vi "Tenney_Main_Temperature_Changer.vi"(0 "Message Queues out":T2, 1 "Elapsed Time (min) Ref":refnum<vi>, 3 "Loop Count Ref":refnum<vi>, 5 "Debug":bool, 7 "Enable Arrays":bool=TRUE, 9 "Tenney Array":refnum<vi>, 11 "error in":errorcluster, 12 "Tenney IP Address":string="10.2.0.248", 13 "Connect Tenney Ref":refnum<vi>, 14 "Data Array":refnum<vi>) -> (15 "error out":errorcluster)   [LabVIEW 2023]
uses:
  Message Queue/All Message Queues.ctl
  Message Queue/Message Cluster.ctl
  Drivers/Tidal Engineering/Type Definitions/Tenney Environmental Chamber Data.ctl
  <vilib>/NI/Modbus Library/API/Master/Modbus Master.lvclass
  Drivers/Tidal Engineering/Type Definitions/Tenney Modbus Registers.ctl
  Drivers/Tidal Engineering/Type Definitions/Tenney Chamber Status.ctl
  controls/Tenney Temperature Limits.ctl
  Drivers/Viasala Indigo 520/Type Definitions/Viasala Indigo 520 Data.ctl
  Message Queue/Enqueue Message (Single).vi
  Message Queue/Tenney Message Queue.lvlib
panel:
  out "Connect Tenney Counter":dbl
  out "10 Minute Data Array Output":dbl[][](array[numeric])
  out "Elapsed Time (min)":dbl caption="Elapsed Time (s)"
  out "Set Chamber Status":dbl
  out "appended array":string[](array[string])
  out "Tenney Environmental Chamber Data Output":T1
  out "Humidity Counter":dbl
  out "Frequency Counter":dbl
  out "Temp Counter":dbl
  out "Loop Count":i32
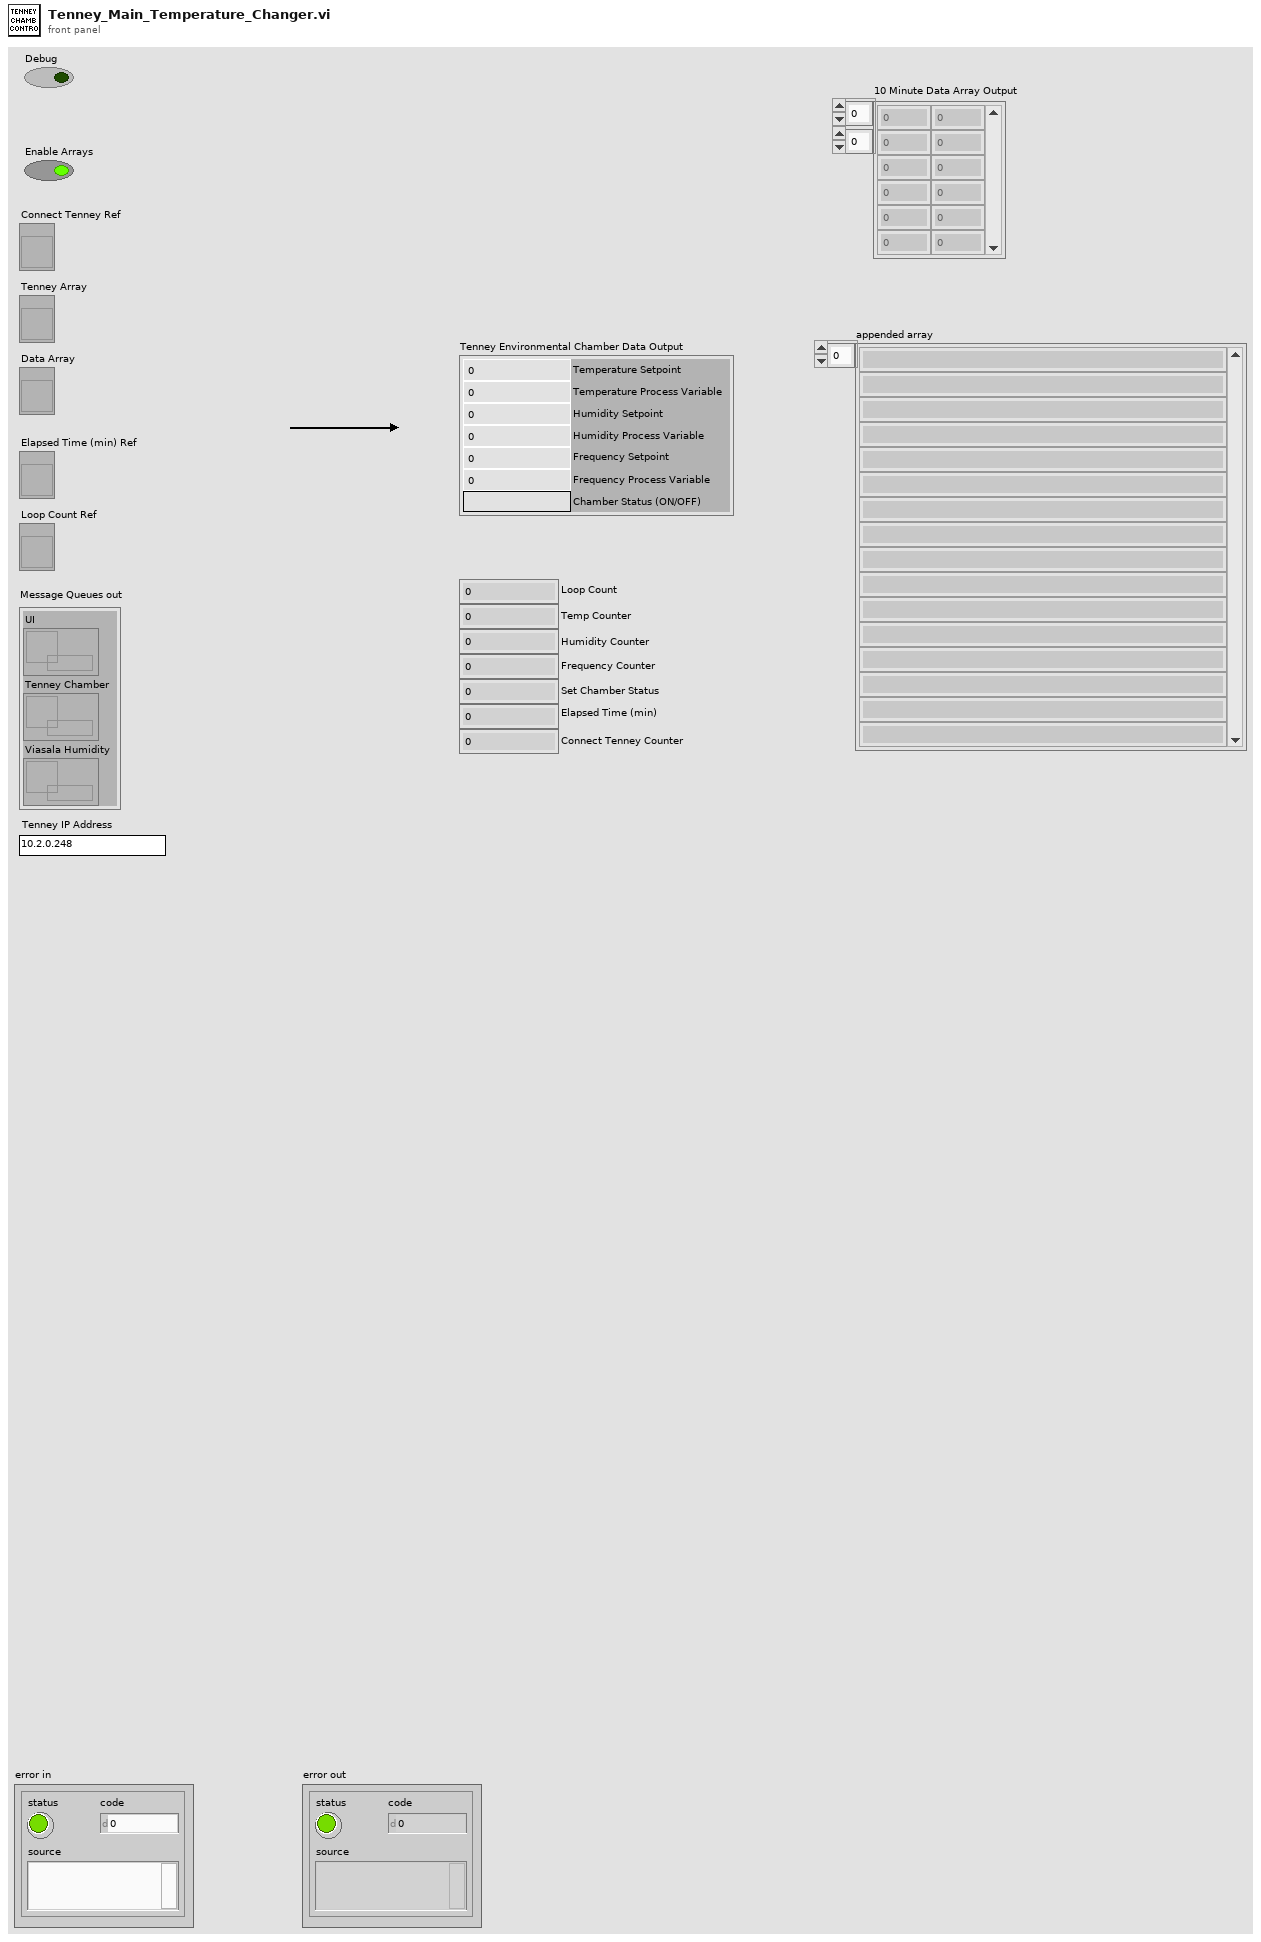
[diagram p1: front panel]
types:
  T1 = typedef "Tenney Environmental Chamber Data.ctl" = cluster{"Temperature Setpoint":dbl, "Temperature Process Variable":dbl, "Humidity Setpoint":dbl, "Humidity Process Variable":dbl, "Frequency Setpoint":dbl, "Frequency Process Variable":dbl, "Chamber Status (ON/OFF)":string}
  T2 = typedef "Tenney Message Queue.lvlib/All Message Queues.ctl" = cluster{"UI":refnum<queue>, "Tenney Chamber":refnum<queue>, "Viasala Humidity":refnum<queue>}
  T3 = typedef "Tenney Chamber Status.ctl" = enum16{"OFF", "ON"}
  T4 = typedef "Tenney Temperature Limits.ctl" = cluster{"Target Temperature Upper limit":dbl, "Target Temperature Lower limit":dbl, "Target Humidity Lower limit":dbl, "Target Humidity Upper limit":dbl, "Chamber Temperature Upper limit":dbl, "Chamber Temperature Lower limit":dbl, "Chamber Humidity Lower limit":dbl, "Chamber Humidity Upper limit":dbl, "Chamber Adjustment Increment (F)":dbl, "Chamber Adjustment Interval (Minutes)":dbl, "Chamber Adjustment Increment (%)":dbl, "Chamber Adjustment Interval Fast (Minutes)":dbl}
  T5 = typedef "Viasala Indigo 520 Data.ctl" = cluster{"Temperature Probe 1":dbl, "Humidity Probe 1":dbl, "Temperature Probe 2":dbl, "Humidity Probe 2":dbl}
  T6 = typedef "Tenney Modbus Registers.ctl" = u16
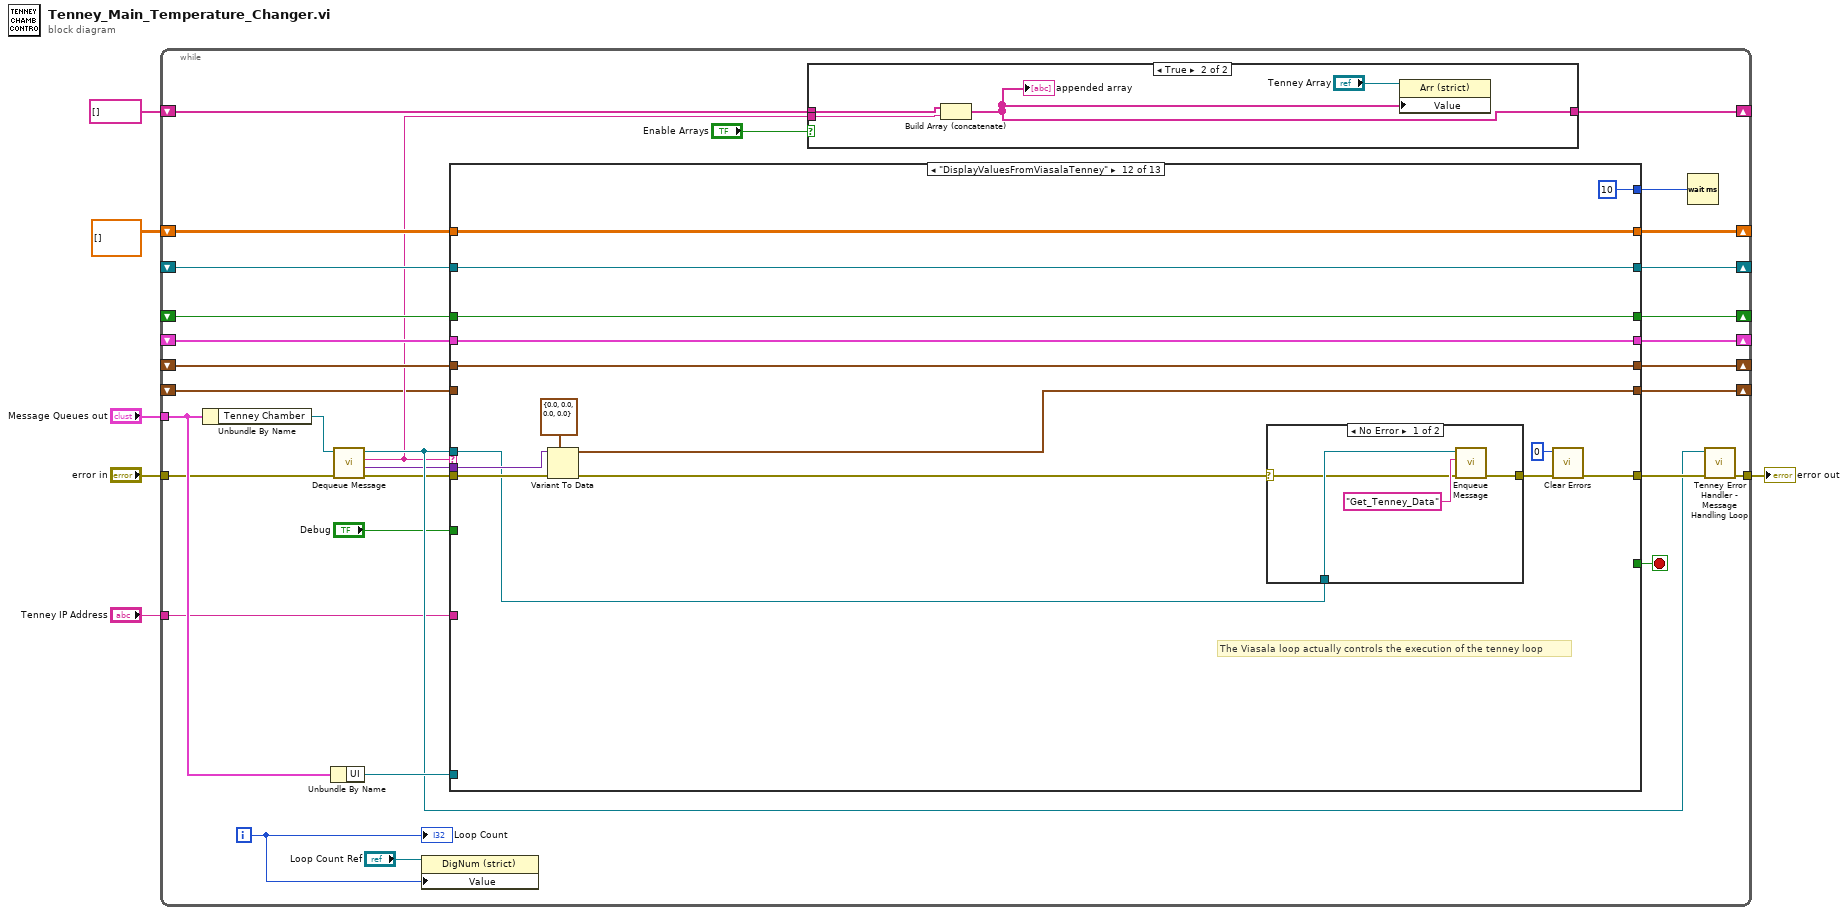
[diagram p0: block diagram]
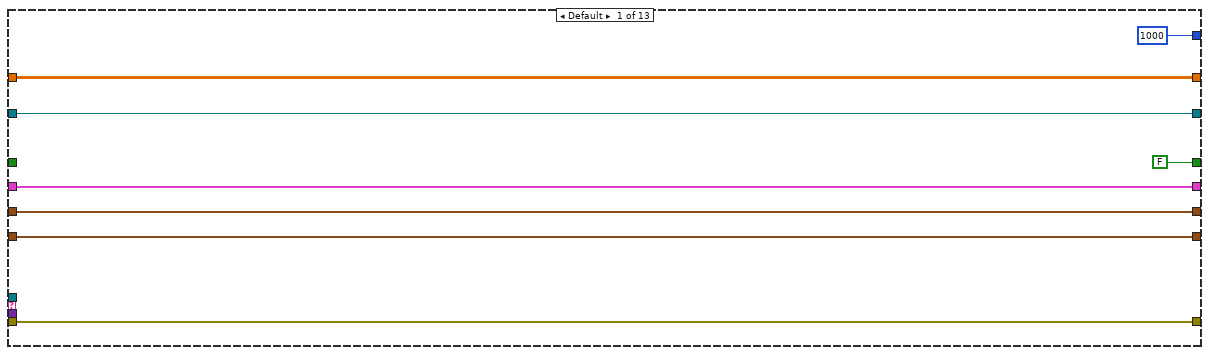
[diagram p3: hidden frame]
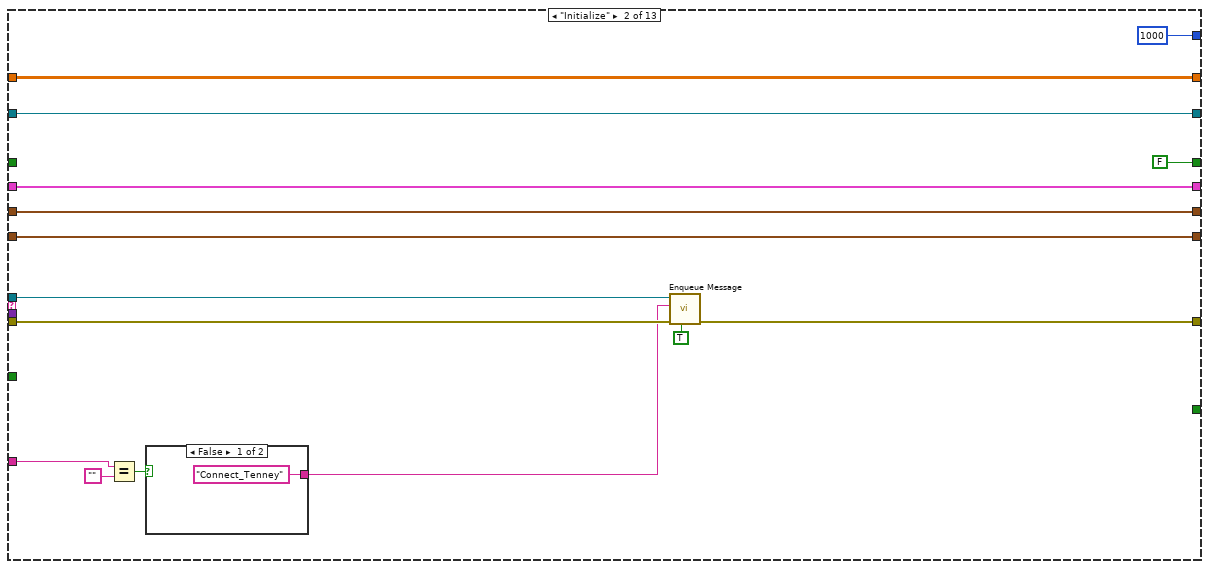
[diagram p4: hidden frame]
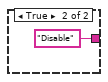
[diagram p5: hidden frame]
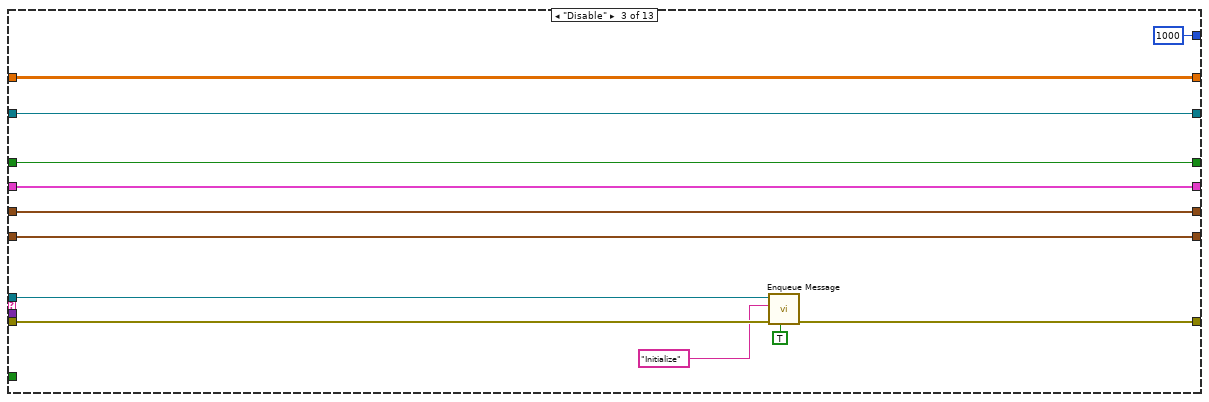
[diagram p6: hidden frame]
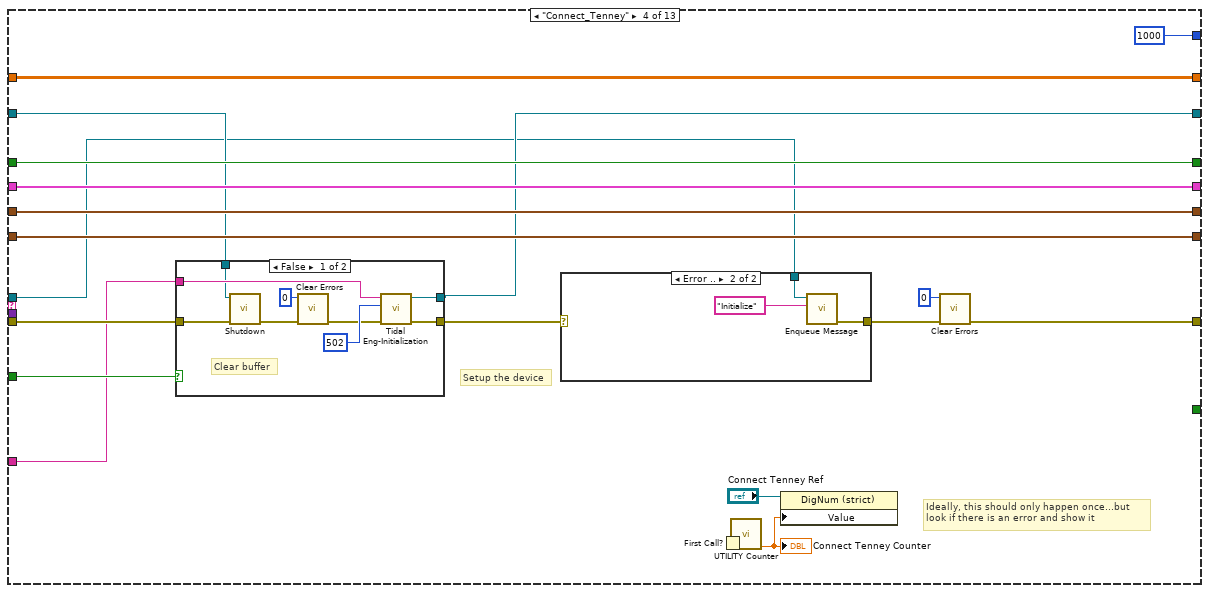
[diagram p7: hidden frame]
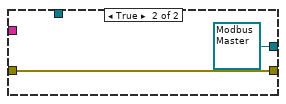
[diagram p8: hidden frame]
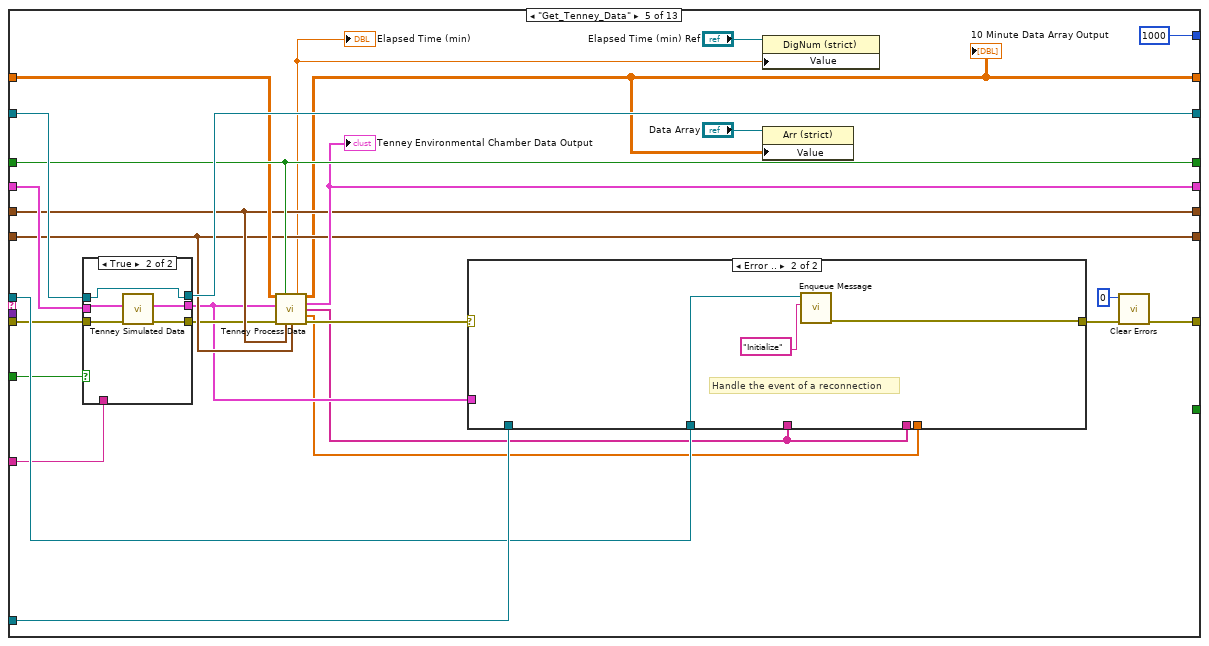
[diagram p10: hidden frame]
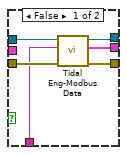
[diagram p11: hidden frame]
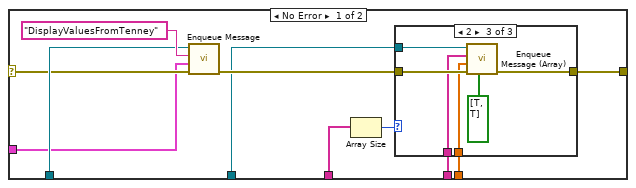
[diagram p12: hidden frame]
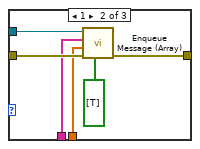
[diagram p14: hidden frame]
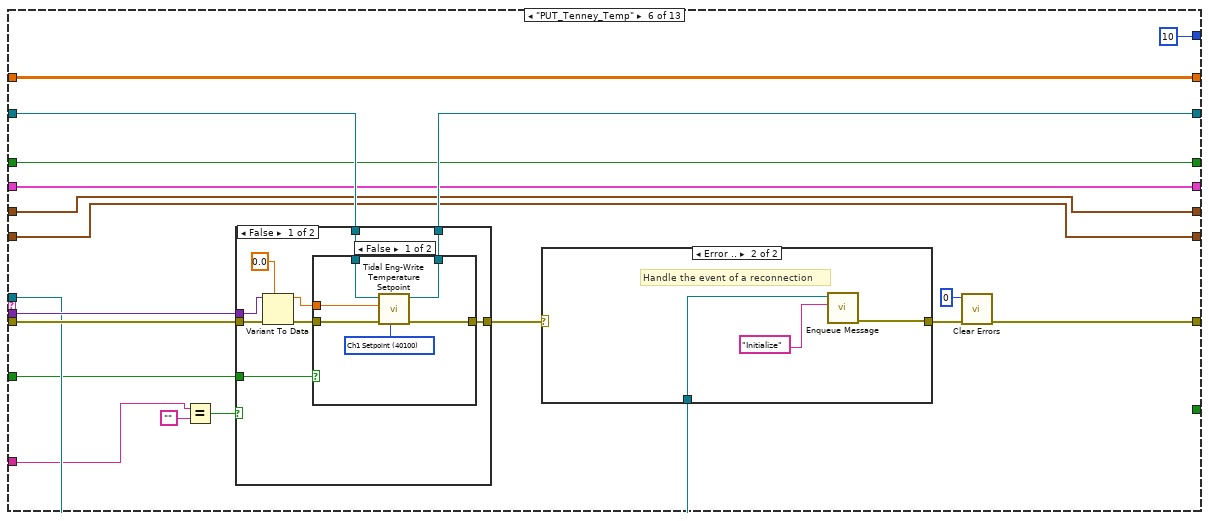
[diagram p15: hidden frame]
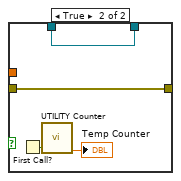
[diagram p16: hidden frame]
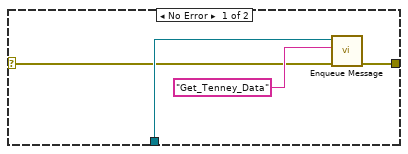
[diagram p18: hidden frame]
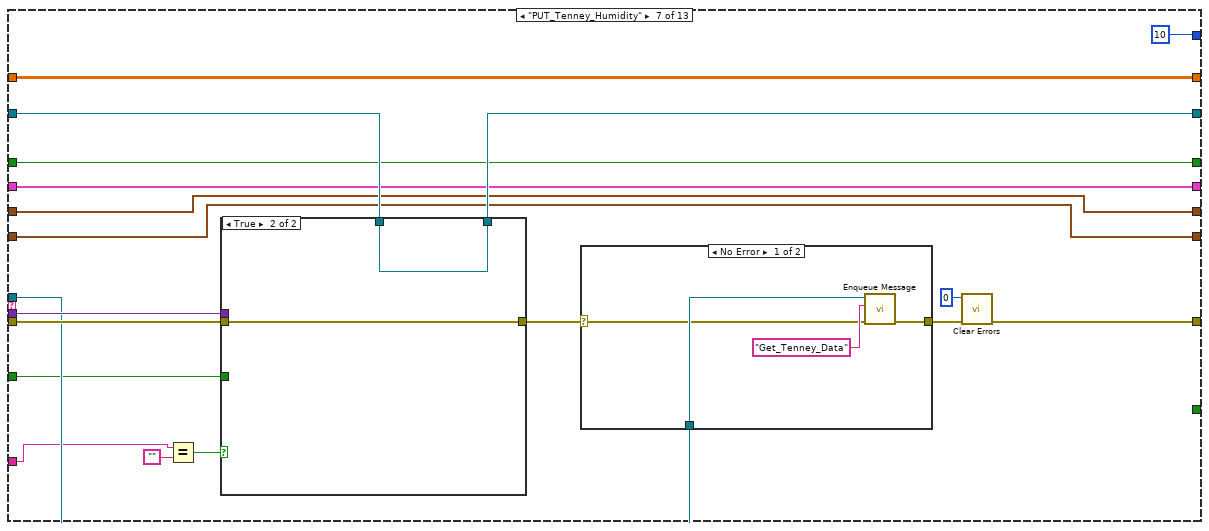
[diagram p19: hidden frame]
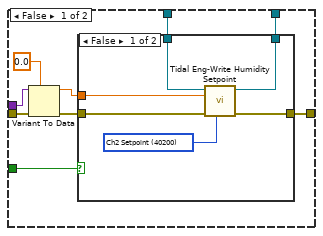
[diagram p20: hidden frame]
diagram:
  n1 = while {
    tunnel: "Message Queues out" -> [w34]
    tunnel: "error in" -> [w30]
    tunnel: [w36] -> w5
    shift-right: [w27] -> _
    shift-left: _ -> [w26]
    shift-right: [w25] -> _
    shift-left: _ -> [w24]
    shift-right: [w22] -> _
    shift-left: dbl[][] [] ("10 Minute Data Array Input") -> [w23]
    shift-right: [w21] -> _
    shift-left: _ -> [w20]
    shift-right: [w18] -> _
    shift-left: _ -> [w17]
    shift-right: [w15] -> _
    shift-left: string[] [] -> [w16]
    shift-right: [w12] -> _
    shift-left: _ -> [w11]
    tunnel: "Tenney IP Address" -> [w7]
    i -> [w10]
    stop <- w37 stop-if-true
    n2 = Unbundle By Name(w34) -> ("Tenney Chamber"=w32:refnum<queue>)
    n3 = Unbundle By Name(w34) -> ("UI"=w33:refnum<queue>)
    n4 = call "Dequeue Message.vi"("error in (no error)"=w30, "Message Queue"=w32) -> ("error out"=w29:errorcluster, "Message Data"=w28:variant, "Message"=w14:string, "dup Message Queue"=w31:refnum<queue>)  [unwired: 6 in]
    n5 = property class="DigNum (strict)"(reference="Loop Count Ref", "Value"=w10) -> ()  [unwired: 1 in, 2 out]
    n6 = case shown="\"DisplayValuesFromViasalaTenney\"" w14 {
      tunnel: w29 -> [w43 w58 w71 w98 w137 w196 w243 w290 w337 w385 w414 w436 w444]
      tunnel: [w43 w57 w70 w87 w121 w194 w241 w288 w336 w383 w412 w434 w453] -> w35
      tunnel: [_ _ _ _ _ _ _ _ _ _ _ _ TRUE] -> w37
      tunnel: w31 -> [_ w59 w69 w86 w138 w193 w240 w287 w335 w380 w409 w431 w455]
      tunnel: w33 -> [_ _ _ _ w139 _ _ _ _ _ _ _ _]
      tunnel: w28 -> [_ _ _ _ _ w195 w242 w289 w325 w384 w413 w435 _]
      tunnel: "Debug" -> [_ _ _ w97 w136 w192 w239 w284 w332 _ _ _ w451]
      tunnel: [w50 w65 w77 w89 w134 w190 w237 w285 w333 w379 w408 w430 w452] -> w27
      tunnel: w26 -> [w50 w65 w77 w88 w135 w191 w238 w286 w334 w379 w408 w430 w452]
      tunnel: [FALSE FALSE w76 w96 w133 w189 w236 w283 w331 w377 w402 w425 w450] -> w25
      tunnel: w24 -> [_ _ w76 w96 w133 w189 w236 w283 w331 _ w402 w425 w450]
      tunnel: w23 -> [w48 w63 w79 w95 w132 w188 w235 w282 w330 w376 w406 w428 w449]
      tunnel: [w48 w63 w79 w95 w122 w188 w235 w282 w330 w376 w406 w428 w449] -> w22
      tunnel: [w47 w62 w75 w94 w131 w187 w234 w281 w329 w375 w405 w427 w448] -> w21
      tunnel: w20 -> [w47 w62 w75 w94 w130 w187 w234 w281 w329 w375 w405 w427 w448]
      tunnel: [u32 1000 ("millisecond multiple") u32 1000 ("millisecond multiple") u32 1000 ("millisecond multiple") u32 1000 ("millisecond multiple") u32 1000 ("millisecond multiple") u32 10 ("millisecond multiple") u32 10 ("millisecond multiple") u32 10 ("millisecond multiple") u32 10 ("millisecond multiple") u32 10 ("millisecond multiple") u32 10 ("millisecond multiple") u32 10 ("millisecond multiple") u32 10 ("millisecond multiple")] -> w19
      tunnel: [w45 w60 w74 w92 w128 w185 w232 w279 w327 w373 w401 w424 w446] -> w18
      tunnel: w17 -> [w45 w60 w74 w92 w128 w185 w232 w279 w327 w373 _ w424 w446]
      tunnel: [w44 w55 w73 w91 w127 w184 w231 w278 w326 w372 w400 w422 w445] -> w12
      tunnel: w11 -> [w44 w55 w73 w91 w127 w184 w231 w278 w326 w372 w400 _ w445]
      tunnel: w7 -> [_ w52 _ w90 w126 w182 w226 w273 w320 w370 _ _ _]
      frame Default {
      }
      frame "Initialize" {
        n7 = Equal?(x=w52, y="") -> (x = y?=w54:bool)
        n8 = case shown="False" w54 {
          tunnel: ["Connect_Tenney" ("Message") "Disable" ("Message")] -> w51
          frame False {
          }
          frame True {
          }
        }
        n9 = call-poly "Enqueue Message.vi"("Priority Message? (F)"=TRUE, "error in (no error)"=w58, "Message"=w51, "Message Queue"=w59) -> ("error out"=w57:errorcluster)  [unwired: 6 in, 1 out]
      }
      frame "Disable" {
        n10 = call-poly "Enqueue Message.vi"("Priority Message? (F)"=TRUE, "error in (no error)"=w71, "Message"="Initialize", "Message Queue"=w69) -> ("error out"=w70:errorcluster)  [unwired: 6 in, 1 out]
      }
      frame "Connect_Tenney" {
        # "Setup the device"
        # "Ideally, this should only happen once...but\nlook if there is an error and show it"
        n11 = case shown="False" w97 {
          tunnel: w98 -> [w103 w109]
          tunnel: [w107 w109] -> w81
          tunnel: [w106 refnum<class "Modbus Master.lvclass"> refnum ("Modbus Master out")] -> w89
          tunnel: w90 -> [w104 _]
          tunnel: w88 -> [w102 _]
          frame False {
            # "Clear buffer"
            n12 = call-dynamic "Shutdown.vi"("error in"=w103, "Modbus master in"=w102) -> ("error out"=w101:errorcluster)  [unwired: 9 in]
            n13 = call <vilib>:"Clear Errors.vi"("error in (no error)"=w101, "specific error code to clear (0: all)"=0) -> ("error out"=w100:errorcluster)  [unwired: 4 in, 1 out]
            n14 = call "Tidal Eng-Initialization.vi"("error in (no error)"=w100, "Remote Port"=u16 502, "IP Address"=w104) -> ("error out"=w107:errorcluster, "Modbus Master out"=w106:refnum<class "Modbus Master.lvclass">)  [unwired: 7 in]
          }
          frame True {
          }
        }
        n15 = case shown="Error .." w81 {
          selector: w81 -> [w110 _]
          tunnel: w86 -> [_ w112]
          tunnel: [w110 w111] -> w80
          frame No Error {
          }
          frame Error {
            n16 = call-poly "Enqueue Message.vi"("Message"="Initialize", "Message Queue"=w112) -> ("error out"=w111:errorcluster)  [unwired: 8 in, 1 out]
          }
        }
        n17 = First Call?() -> (First Call?: T/F=w84:bool)
        n18 = call "UTILITY Counter.vi"("Reset"=w84) -> ("Count"=w85:dbl)  [unwired: 10 in]
        "Connect Tenney Counter" <- w85
        n19 = property class="DigNum (strict)"(reference="Connect Tenney Ref", "Value"=w85) -> ()  [unwired: 1 in, 2 out]
        n20 = call <vilib>:"Clear Errors.vi"("error in (no error)"=w80, "specific error code to clear (0: all)"=0) -> ("error out"=w87:errorcluster)  [unwired: 4 in, 1 out]
      }
      frame "Get_Tenney_Data" {
        n21 = case shown="True" w136 {
          tunnel: w137 -> [w145 w150]
          tunnel: [w144 w149] -> w120
          tunnel: [w143 w147] -> w118
          tunnel: w135 -> [w142 w148]
          tunnel: [w141 w148] -> w134
          tunnel: w130 -> [_ w146]
          tunnel: w126 -> [w140 _]
          frame False {
            n22 = call "Tidal Eng-Modbus Data.vi"("error in (no error)"=w145, "IP Address"=w140, "Modbus master in"=w142) -> ("error out"=w144:errorcluster, "Tenney Environmental Chamber Data Output"=w143:T1, "Modbus master out"=w141:refnum<class "Modbus Master.lvclass">)  [unwired: 5 in, 1 out]
          }
          frame True {
            n23 = call "Tenney Simulated Data.vi"("error in (no error)"=w150, "Tenney Environmental Chamber Data Input"=w146) -> ("error out"=w149:errorcluster, "Tenney Environmental Chamber Data Output"=w147:T1)  [unwired: 8 in]
          }
        }
        n24 = call "Tenney Process Data.vi"("10 Minute Data Array Input"=w132, "Auto Control Input"=w133, "Tenney Environmental Chamber Data Input"=w118, "error in (no error)"=w120, "Temperature Limits"=w128, "Viasala Data Output"=w127) -> ("Elapsed Time (min)"=w124:dbl, "10 Minute Data Array Output"=w122:dbl[][], "Tenney Environmental Chamber Data Output"=w131:T1, "Output CMD"=w116:string[], "Data CMD"=w117:dbl[], "error out"=w119:errorcluster)  [unwired: 4 in]
        "Tenney Environmental Chamber Data Output" <- w131
        "Elapsed Time (min)" <- w124
        "10 Minute Data Array Output" <- w122
        n25 = case shown="Error .." w119 {
          selector: w119 -> [w159 _]
          tunnel: w139 -> [w160 _]
          tunnel: [w156 w177] -> w114
          tunnel: w138 -> [w155 w175]
          tunnel: w118 -> [w158 _]
          tunnel: w116 -> [w154 _]
          tunnel: w117 -> [w153 _]
          tunnel: w116 -> [w151 _]
          frame No Error {
            n26 = call-poly "Enqueue Message.vi"("error in (no error)"=w159, "Message Data"=w158, "Message"="DisplayValuesFromTenney", "Message Queue"=w160) -> ("error out"=w157:errorcluster)  [unwired: 6 in, 1 out]
            n27 = Array Size(array=w151) -> (size(s)=w152:i32)
            n28 = case shown="2" w152 {
              tunnel: w157 -> [w162 w168 w173]
              tunnel: [w162 w167 w172] -> w156
              tunnel: w155 -> [_ w166 w171]
              tunnel: w154 -> [_ w165 w170]
              tunnel: w153 -> [_ w164 w169]
              frame Default {
              }
              frame 1 {
                n29 = call "Enqueue Message (Array).vi"("Priority Message? Array"=bool[] [TRUE], "error in (no error)"=w168, "Message Data Array"=w164, "Message Array"=w165, "Message Queue"=w166) -> ("error out"=w167:errorcluster)  [unwired: 5 in, 1 out]
              }
              frame 2 {
                n30 = call "Enqueue Message (Array).vi"("Priority Message? Array"=bool[] [TRUE, TRUE], "error in (no error)"=w173, "Message Data Array"=w169, "Message Array"=w170, "Message Queue"=w171) -> ("error out"=w172:errorcluster)  [unwired: 5 in, 1 out]
              }
            }
          }
          frame Error {
            # "Handle the event of a reconnection"
            n31 = call-poly "Enqueue Message.vi"("Message"="Initialize", "Message Queue"=w175) -> ("error out"=w177:errorcluster)  [unwired: 8 in, 1 out]
          }
        }
        n32 = property class="DigNum (strict)"(reference="Elapsed Time (min) Ref", "Value"=w124) -> ()  [unwired: 1 in, 2 out]
        n33 = property class="Arr (strict)"(reference="Data Array", "Value"=w122) -> ()  [unwired: 1 in, 2 out]
        n34 = call <vilib>:"Clear Errors.vi"("error in (no error)"=w114, "specific error code to clear (0: all)"=0) -> ("error out"=w121:errorcluster)  [unwired: 4 in, 1 out]
      }
      frame "PUT_Tenney_Temp" {
        n35 = Equal?(x=w182, y="") -> (x = y?=w178:bool)
        n36 = case shown="False" w178 {
          tunnel: w196 -> [w205 w216]
          tunnel: w195 -> [w204 _]
          tunnel: w192 -> [w203 _]
          tunnel: w191 -> [w202 w217]
          tunnel: [w201 w217] -> w190
          tunnel: [w199 w216] -> w179
          frame False {
            n37 = Variant To Data(error in=w205, type=0.0, Variant=w204) -> (data=w197:dbl, error out=w200:errorcluster)
            n38 = case shown="False" w203 {
              tunnel: w200 -> [w211 w215]
              tunnel: [w210 w215] -> w199
              tunnel: w202 -> [w209 w214]
              tunnel: [w208 w214] -> w201
              tunnel: w197 -> [w207 _]
              frame False {
                w206 = T6 40100 items=["Ch1 Setpoint"=40100, "Ch1 Process Variable"=40103, "Ch2 Setpoint"=40200, "Ch2 Process Variable"=40203, "Ch3 Setpoint"=40300, "Ch3 Process Variable"=40303, "All Events Mask"=40500, "Run State"=40600] ("Temperature Setpoint")
                n39 = call "Tidal Eng-Write Temperature Setpoint.vi"("Temperature Setpoint"=w206, "error in (no error)"=w211, "Temperature (°F)"=w207, "Modbus master in"=w209) -> ("error out"=w210:errorcluster, "Modbus master out"=w208:refnum<class "Modbus Master.lvclass">)  [unwired: 6 in]
              }
              frame True {
                n40 = First Call?() -> (First Call?: T/F=w212:bool)
                n41 = call "UTILITY Counter.vi"("Reset"=w212) -> ("Count"=→"Temp Counter":dbl)  [unwired: 10 in]
              }
            }
          }
          frame True {
          }
        }
        n42 = case shown="Error .." w179 {
          selector: w179 -> [w218 _]
          tunnel: [w220 w224] -> w180
          tunnel: w193 -> [w219 w222]
          frame No Error {
            n43 = call-poly "Enqueue Message.vi"("error in (no error)"=w218, "Message"="Get_Tenney_Data", "Message Queue"=w219) -> ("error out"=w220:errorcluster)  [unwired: 7 in, 1 out]
          }
          frame Error {
            # "Handle the event of a reconnection"
            n44 = call-poly "Enqueue Message.vi"("Message"="Initialize", "Message Queue"=w222) -> ("error out"=w224:errorcluster)  [unwired: 8 in, 1 out]
          }
        }
        n45 = call <vilib>:"Clear Errors.vi"("error in (no error)"=w180, "specific error code to clear (0: all)"=0) -> ("error out"=w194:errorcluster)  [unwired: 4 in, 1 out]
      }
      frame "PUT_Tenney_Humidity" {
        n46 = Equal?(x=w226, y="") -> (x = y?=w225:bool)
        n47 = case shown="True" w225 {
          tunnel: w243 -> [w252 w263]
          tunnel: w242 -> [w251 _]
          tunnel: w239 -> [w247 _]
          tunnel: w238 -> [w246 w264]
          tunnel: [w245 w264] -> w237
          tunnel: [w244 w263] -> w228
          frame False {
            n48 = Variant To Data(error in=w252, type=0.0, Variant=w251) -> (data=w248:dbl, error out=w250:errorcluster)
            n49 = case shown="False" w247 {
              tunnel: w250 -> [w258 w262]
              tunnel: [w257 w262] -> w244
              tunnel: w248 -> [w256 _]
              tunnel: w246 -> [w255 w261]
              tunnel: [w254 w261] -> w245
              frame False {
                w253 = T6 40200 items=["Ch1 Setpoint"=40100, "Ch1 Process Variable"=40103, "Ch2 Setpoint"=40200, "Ch2 Process Variable"=40203, "Ch3 Setpoint"=40300, "Ch3 Process Variable"=40303, "All Events Mask"=40500, "Run State"=40600] ("Temperature Setpoint")
                n50 = call "Tidal Eng-Write Humidity Setpoint.vi"("Temperature Setpoint"=w253, "error in (no error)"=w258, "Humidity (%)"=w256, "Modbus master in"=w255) -> ("error out"=w257:errorcluster, "Modbus master out"=w254:refnum<class "Modbus Master.lvclass">)  [unwired: 6 in]
              }
              frame True {
                n51 = First Call?() -> (First Call?: T/F=w259:bool)
                n52 = call "UTILITY Counter.vi"("Reset"=w259) -> ("Count"=→"Humidity Counter":dbl)  [unwired: 10 in]
              }
            }
          }
          frame True {
          }
        }
        n53 = case shown="No Error" w228 {
          selector: w228 -> [w265 _]
          tunnel: [w267 w271] -> w229
          tunnel: w240 -> [w266 w269]
          frame No Error {
            n54 = call-poly "Enqueue Message.vi"("error in (no error)"=w265, "Message"="Get_Tenney_Data", "Message Queue"=w266) -> ("error out"=w267:errorcluster)  [unwired: 7 in, 1 out]
          }
          frame Error {
            # "Handle the event of a reconnection"
            n55 = call-poly "Enqueue Message.vi"("Message"="Initialize", "Message Queue"=w269) -> ("error out"=w271:errorcluster)  [unwired: 8 in, 1 out]
          }
        }
        n56 = call <vilib>:"Clear Errors.vi"("error in (no error)"=w229, "specific error code to clear (0: all)"=0) -> ("error out"=w241:errorcluster)  [unwired: 4 in, 1 out]
      }
      frame "PUT_Tenney_Frequency" {
        n57 = Equal?(x=w273, y="") -> (x = y?=w272:bool)
        n58 = case shown="False" w272 {
          tunnel: w290 -> [w299 w310]
          tunnel: w289 -> [w298 _]
          tunnel: w286 -> [w296 w311]
          tunnel: [w295 w311] -> w285
          tunnel: w284 -> [w292 _]
          tunnel: [w291 w310] -> w275
          frame False {
            n59 = Variant To Data(error in=w299, type=0.0, Variant=w298) -> (data=w293:dbl, error out=w297:errorcluster)
            n60 = case shown="False" w292 {
              tunnel: w297 -> [w305 w308]
              tunnel: [w304 w308] -> w291
              tunnel: w296 -> [w303 w309]
              tunnel: [w302 w309] -> w295
              tunnel: w293 -> [w301 _]
              frame False {
                w300 = T6 40300 items=["Ch1 Setpoint"=40100, "Ch1 Process Variable"=40103, "Ch2 Setpoint"=40200, "Ch2 Process Variable"=40203, "Ch3 Setpoint"=40300, "Ch3 Process Variable"=40303, "All Events Mask"=40500, "Run State"=40600] ("Temperature Setpoint")
                n61 = call "Tidal Eng-Write Frequency Setpoint.vi"("Temperature Setpoint"=w300, "error in (no error)"=w305, "Frequency (Hz)"=w301, "Modbus master in"=w303) -> ("error out"=w304:errorcluster, "Modbus master out"=w302:refnum<class "Modbus Master.lvclass">)  [unwired: 6 in]
              }
              frame True {
                n62 = First Call?() -> (First Call?: T/F=w306:bool)
                n63 = call "UTILITY Counter.vi"("Reset"=w306) -> ("Count"=→"Frequency Counter":dbl)  [unwired: 10 in]
              }
            }
          }
          frame True {
          }
        }
        n64 = case shown="Error .." w275 {
          selector: w275 -> [w312 _]
          tunnel: [w314 w318] -> w276
          tunnel: w287 -> [w313 w316]
          frame No Error {
            n65 = call-poly "Enqueue Message.vi"("error in (no error)"=w312, "Message"="Get_Tenney_Data", "Message Queue"=w313) -> ("error out"=w314:errorcluster)  [unwired: 7 in, 1 out]
          }
          frame Error {
            # "Handle the event of a reconnection"
            n66 = call-poly "Enqueue Message.vi"("Message"="Initialize", "Message Queue"=w316) -> ("error out"=w318:errorcluster)  [unwired: 8 in, 1 out]
          }
        }
        n67 = call <vilib>:"Clear Errors.vi"("error in (no error)"=w276, "specific error code to clear (0: all)"=0) -> ("error out"=w288:errorcluster)  [unwired: 4 in, 1 out]
      }
      frame "PUT_Chamber_Status" {
        n68 = Equal?(x=w320, y="") -> (x = y?=w319:bool)
        n69 = case shown="True" w319 {
          tunnel: w337 -> [w346 w360]
          tunnel: w334 -> [w344 w361]
          tunnel: [w343 w361] -> w333
          tunnel: w332 -> [w342 _]
          tunnel: w325 -> [w340 _]
          tunnel: [w338 w360] -> w322
          frame False {
            n70 = Variant To Data(error in=w346, type=Tenney_Chamber_Status."OFF" ("Chamber Status"), Variant=w340) -> (data=w339:T3, error out=w345:errorcluster)
            n71 = case shown="False" w342 {
              tunnel: w345 -> [w351 w358]
              tunnel: [w350 w358] -> w338
              tunnel: w344 -> [w353 w359]
              tunnel: [w352 w359] -> w343
              tunnel: w339 -> [w348 _]
              frame False {
                w349 = T6 40600 items=["Ch1 Setpoint"=40100, "Ch1 Process Variable"=40103, "Ch2 Setpoint"=40200, "Ch2 Process Variable"=40203, "Ch3 Setpoint"=40300, "Ch3 Process Variable"=40303, "All Events Mask"=40500, "Run State"=40600] ("Modbus Registers")
                n72 = case shown="\"ON\"" w348 {
                  tunnel: [u16 0 ("register to write") u16 3 ("register to write")] -> w347
                  frame "OFF", Default {
                  }
                  frame "ON" {
                  }
                }
                n73 = call-dynamic "Write Single Holding Register.vi"("error in"=w351, "register to write"=w347, "address"=w349, "Modbus master in"=w353) -> ("error out"=w350:errorcluster, "Modbus master out"=w352:refnum<class "Modbus Master.lvclass">)  [unwired: 6 in]
              }
              frame True {
                n74 = First Call?() -> (First Call?: T/F=w356:bool)
                n75 = call "UTILITY Counter.vi"("Reset"=w356) -> ("Count"=→"Set Chamber Status":dbl)  [unwired: 10 in]
              }
            }
          }
          frame True {
          }
        }
        n76 = case shown="Error .." w322 {
          selector: w322 -> [w362 _]
          tunnel: [w364 w368] -> w323
          tunnel: w335 -> [w363 w366]
          frame No Error {
            n77 = call-poly "Enqueue Message.vi"("error in (no error)"=w362, "Message"="Get_Tenney_Data", "Message Queue"=w363) -> ("error out"=w364:errorcluster)  [unwired: 7 in, 1 out]
          }
          frame Error {
            # "Handle the event of a reconnection"
            n78 = call-poly "Enqueue Message.vi"("Message"="Initialize", "Message Queue"=w366) -> ("error out"=w368:errorcluster)  [unwired: 8 in, 1 out]
          }
        }
        n79 = call <vilib>:"Clear Errors.vi"("error in (no error)"=w323, "specific error code to clear (0: all)"=0) -> ("error out"=w336:errorcluster)  [unwired: 4 in, 1 out]
      }
      frame "Tenney_Enable_Auto_Control" {
        n80 = Equal?(x=w370, y="") -> (x = y?=w369:bool)
        n81 = case shown="False" w369 {
          tunnel: w385 -> [w390 w391]
          tunnel: w384 -> [w389 _]
          tunnel: [w388 w391] -> w378
          tunnel: [w386 FALSE] -> w377
          frame False {
            n82 = Variant To Data(error in=w390, type=TRUE, Variant=w389) -> (data=w386:bool, error out=w388:errorcluster)
          }
          frame True {
          }
        }
        n83 = case shown="Error .." w378 {
          selector: w378 -> [w393 _]
          tunnel: [w395 w399] -> w381
          tunnel: w380 -> [w394 w397]
          frame No Error {
            n84 = call-poly "Enqueue Message.vi"("error in (no error)"=w393, "Message"="Get_Tenney_Data", "Message Queue"=w394) -> ("error out"=w395:errorcluster)  [unwired: 7 in, 1 out]
          }
          frame Error {
            # "Handle the event of a reconnection"
            n85 = call-poly "Enqueue Message.vi"("Message"="Initialize", "Message Queue"=w397) -> ("error out"=w399:errorcluster)  [unwired: 8 in, 1 out]
          }
        }
        n86 = call <vilib>:"Clear Errors.vi"("error in (no error)"=w381, "specific error code to clear (0: all)"=0) -> ("error out"=w383:errorcluster)  [unwired: 4 in, 1 out]
      }
      frame "Update_Temp_Limits" {
        n87 = Variant To Data(error in=w414, type=T4 {"Target Temperature Upper limit"=68.0, "Target Temperature Lower limit"=67.0, "Target Humidity Lower limit"=48.5, "Target Humidity Upper limit"=51.5, "Chamber Temperature Upper limit"=73.0, "Chamber Temperature Lower limit"=63.0, "Chamber Humidity Lower limit"=40.0, "Chamber Humidity Upper limit"=60.0, "Chamber Adjustment Increment (F)"=0.1, "Chamber Adjustment Interval (Minutes)"=10.0, "Chamber Adjustment Increment (%)"=0.1, "Chamber Adjustment Interval Fast (Minutes)"=5.0} ("Temperature Limits"), Variant=w413) -> (data=w401:T4, error out=w407:errorcluster)
        n88 = case shown="Error .." w407 {
          selector: w407 -> [w415 _]
          tunnel: [w417 w421] -> w410
          tunnel: w409 -> [w416 w419]
          frame No Error {
            n89 = call-poly "Enqueue Message.vi"("error in (no error)"=w415, "Message"="Get_Tenney_Data", "Message Queue"=w416) -> ("error out"=w417:errorcluster)  [unwired: 7 in, 1 out]
          }
          frame Error {
            # "Handle the event of a reconnection"
            n90 = call-poly "Enqueue Message.vi"("Message"="Initialize", "Message Queue"=w419) -> ("error out"=w421:errorcluster)  [unwired: 8 in, 1 out]
          }
        }
        n91 = call <vilib>:"Clear Errors.vi"("error in (no error)"=w410, "specific error code to clear (0: all)"=0) -> ("error out"=w412:errorcluster)  [unwired: 4 in, 1 out]
      }
      frame "DisplayValuesFromViasalaTenney" {
        # "The Viasala loop actually controls the execution of the tenney loop"
        n92 = Variant To Data(error in=w436, type=T5 {"Temperature Probe 1"=0.0, "Humidity Probe 1"=0.0, "Temperature Probe 2"=0.0, "Humidity Probe 2"=0.0} ("Viasala Data Output"), Variant=w435) -> (data=w422:T5, error out=w429:errorcluster)
        n93 = case shown="No Error" w429 {
          selector: w429 -> [w437 _]
          tunnel: [w439 w443] -> w432
          tunnel: w431 -> [w438 w441]
          frame No Error {
            n94 = call-poly "Enqueue Message.vi"("error in (no error)"=w437, "Message"="Get_Tenney_Data", "Message Queue"=w438) -> ("error out"=w439:errorcluster)  [unwired: 7 in, 1 out]
          }
          frame Error {
            # "Handle the event of a reconnection"
            n95 = call-poly "Enqueue Message.vi"("Message"="Initialize", "Message Queue"=w441) -> ("error out"=w443:errorcluster)  [unwired: 8 in, 1 out]
          }
        }
        n96 = call <vilib>:"Clear Errors.vi"("error in (no error)"=w432, "specific error code to clear (0: all)"=0) -> ("error out"=w434:errorcluster)  [unwired: 4 in, 1 out]
      }
      frame "Exit" {
        n97 = Release Queue(queue=w455, error in (no error)=w444) -> (error out=w454:errorcluster)  [unwired: 1 in, 2 out]
        n98 = case shown="True" w451 {
          tunnel: w454 -> [w459 w460]
          tunnel: [w458 w460] -> w453
          tunnel: w452 -> [w457 _]
          frame False {
            n99 = call-dynamic "Shutdown.vi"("error in"=w459, "Modbus master in"=w457) -> ("error out"=w458:errorcluster)  [unwired: 9 in]
          }
          frame True {
          }
        }
      }
    }
    n100 = case shown="True" "Enable Arrays" {
      tunnel: w16 -> [w38 w42]
      tunnel: [w38 w39] -> w15
      tunnel: w14 -> [_ w41]
      frame False {
      }
      frame True {
        n101 = Build Array (concatenate)(w42, w41) -> (w39:string[])
        "appended array" <- w39
        n102 = property class="Arr (strict)"(reference="Tenney Array", "Value"=w39) -> ()  [unwired: 1 in, 2 out]
      }
    }
    n103 = Wait (ms)(milliseconds to wait=w19) -> ()  [unwired: 1 out]
    n104 = call "Tenney Error Handler - Message Handling Loop.vi"("error in (no error)"=w35, "Message Queue"=w31) -> ("dup error in"=w36:errorcluster)  [unwired: 8 in, 1 out]
    "Loop Count" <- w10
  }
  "error out" <- w5
